vi "error_bypass.vi"   [LabVIEW 2015]
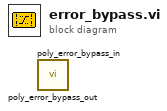
[diagram p0: block diagram]
diagram:
  n1 = call "poly_error_bypass_out.vi"() -> ()  [unwired: 10 in, 2 out]
  n2 = call "poly_error_bypass_in.vi"() -> ()  [unwired: 11 in, 1 out]
